vi "Drive_Globals.vi"() -> ()   [LabVIEW 2019]
uses:
  Subsystems/Drive/Drive_Cluster.ctl
  Subsystems/Drive/Drive_Control_States.ctl
  Subsystems/Drive/Drive_Orientation_States.ctl
panel:
  in  "Set_Heading(deg)":dbl
  in  "Set_Y_Position(in)":dbl
  in  "Set_X_Position(in)":dbl
  in  "Set_Pose":bool
  in  "Zero_Pose":bool
  in  "Azimuth_Motor_Back_Right":dbl
  in  "Azimuth_Motor_Back_Left":dbl
  in  "Azimuth_Motor_Front_Left":dbl
  in  "Azimuth_Motor_Front_Right":dbl
  in  "Drive_Motor_Back_Right":dbl
  in  "Drive_Motor_Back_Left":dbl
  in  "Drive_Motor_Front_Left":dbl
  in  "Drive_Motor_Front_Right":dbl
  in  "Drive_Execute_Ref":string="Drive_Execute_Ref"
  in  "Drive_Set_Ref":string="Drive_Set_Ref"
  in  "Drive_Execute_Notifier":refnum<notifier>
  in  "Drive_Set_Notifier":refnum<notifier>
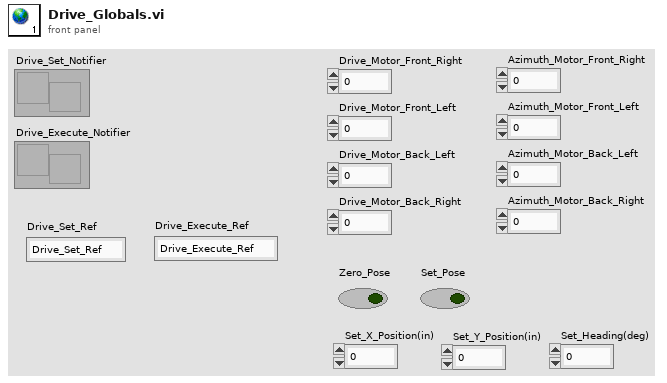
[diagram p1: front panel]
diagram:
